vi "TEST Set Timeout.vi"(8 "error in (no error)":errorcluster) -> (0 "error out":errorcluster)   [LabVIEW 2013, in "TEST JKI State Machine API.lvlib"]
uses:
  TEST JKI State Machine API.lvlib
  <vilib>/addons/_JKI Toolkits/Caraya/classes/Test/Test.lvclass
  source/JKI SM/JKI SM.lvclass
  <vilib>/addons/_JKI Toolkits/Caraya/classes/Assert/Assert.lvclass
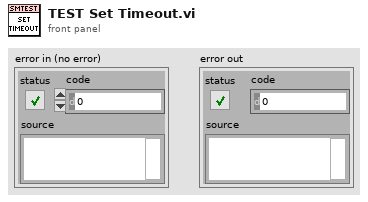
[diagram p1: front panel]
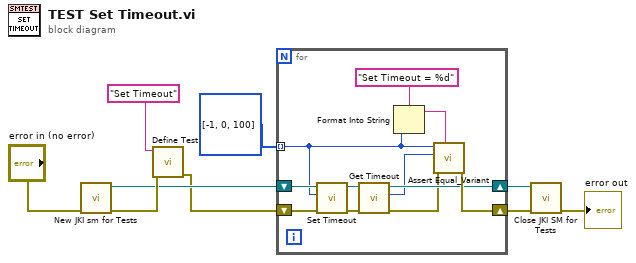
[diagram p0: block diagram]
diagram:
  n1 = call "New JKI sm for Tests.vi"("error in (no error)"="error in (no error)") -> ("error out"=w9:errorcluster, "JKI SM out"=w4:refnum<class "JKI SM.lvclass">)  [unwired: 9 in]
  n2 = call <vilib>:"Define Test.vi"("error in (no error)"=w9, "Label (VI Title)"="Set Timeout") -> ("error out"=w2:errorcluster)  [unwired: 9 in]
  n3 = for {
    tunnel: i32[] [-1, 0, 100] -> [w10] mode=indexing
    shift-right: [w20] -> w6
    shift-left: w2 -> [w15]
    shift-right: [w16] -> w3
    shift-left: w4 -> [w19]
    n4 = call "Set Timeout.vi"("error in (no error)"=w15, "Timeout (ms)"=w10, "JKI SM in"=w19) -> ("error out"=w17:errorcluster, "JKI SM out"=w18:refnum<class "JKI SM.lvclass">)  [unwired: 7 in]
    n5 = call "Get Timeout.vi"("error in (no error)"=w17, "JKI SM in"=w18) -> ("error out"=w14:errorcluster, "Timeout (ms)"=w13:i32, "JKI SM out"=w16:refnum<class "JKI SM.lvclass">)  [unwired: 7 in]
    n6 = Format Into String(format string="Set Timeout = %d" ("Label"), w10) -> (resulting string=w11:string)  [unwired: 2 in, 1 out]
    n7 = call <vilib>:"Assert Equal_Variant.vi"("Label"=w11, "error in (no error)"=w14, "Y"=w13, "X"=w10) -> ("error out"=w20:errorcluster)  [unwired: 7 in]
  }
  n8 = call "Close JKI SM for Tests.vi"("error in (no error)"=w6, "JKI SM in"=w3) -> ("error out"=→"error out":errorcluster)  [unwired: 9 in]
